vi "read serial text data.vi"(8 "error in (no error)":errorcluster, 11 "serial port":refnum<visa-resource-name>) -> (0 "error out":errorcluster, 1 "data read":bool, 2 "serial data":dbl[][](array[numeric]), 3 "VISA resource name out":refnum<visa-resource-name>)   [LabVIEW 2017]
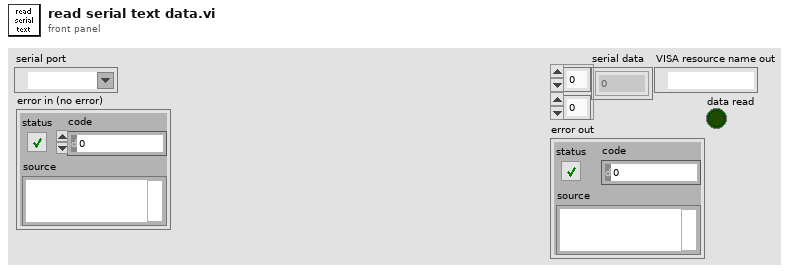
[diagram p1: front panel]
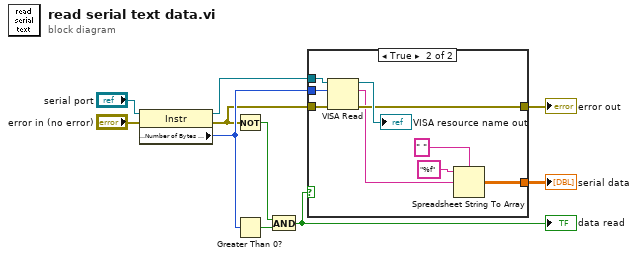
[diagram p0: block diagram]
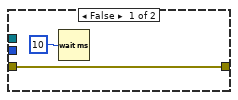
[diagram p2: hidden frame]
diagram:
  n1 = property class="Instr"(reference="serial port", error in="error in (no error)") -> (reference out=w10:refnum<visa-resource-name>, error out=w2:errorcluster, "Serial Settings:Number of Bytes at Serial Port"=w5:u32)
  n2 = Not(x=w2) -> (.not. x?=w1:bool)
  n3 = Greater Than 0?(x=w5) -> (x > 0?=w3:bool)
  n4 = And(x=w1, y=w3) -> (x .and. y?=w4:bool)
  "data read" <- w4
  n5 = case shown="True" w4 {
    tunnel: w5 -> [_ w21]
    tunnel: w10 -> [_ w20]
    tunnel: w2 -> [w12 w19]
    tunnel: [_ w16] -> w7
    tunnel: [w12 w14] -> w6
    frame False {
      n6 = Wait (ms)(milliseconds to wait=u32 10) -> ()  [unwired: 1 out]
    }
    frame True {
      n7 = VISA Read(VISA resource name=w20, byte count=w21, error in (no error)=w19) -> (VISA resource name out=→"VISA resource name out":refnum<visa-resource-name>, read buffer=w13:string, error out=w14:errorcluster)  [unwired: 1 out]
      n8 = Spreadsheet String To Array(delimiter (Tab)=" ", format string="%f", spreadsheet string=w13) -> (array=w16:dbl[][])  [unwired: 1 in]
    }
  }
  "serial data" <- w7
  "error out" <- w6
